vi "process raw data (SubVI).vi"(0 "VISA Refnum in":refnum<visa-resource-name>, 5 "error in (no error)":errorcluster) -> (6 "Raw Data":string, 8 "RSM (Digital)":dbl, 9 "Rain Intensity":dbl(slide) scale=0.0..100.0, 10 "Servo Angle (A)":dbl, 11 "Buzzer Volume (A)":dbl, 12 "Physical Switch State (D)":dbl, 13 "Buzzer Volume":dbl(graph), 14 "VISA Refnum out":refnum<visa-resource-name>, 15 "Servo Angle":dbl(graph), 16 "Rain \nDetected?":bool, 17 "RSM (Analog)":dbl, 18 "Force\nClose?":bool, 19 "error out":errorcluster)   [LabVIEW 2026]
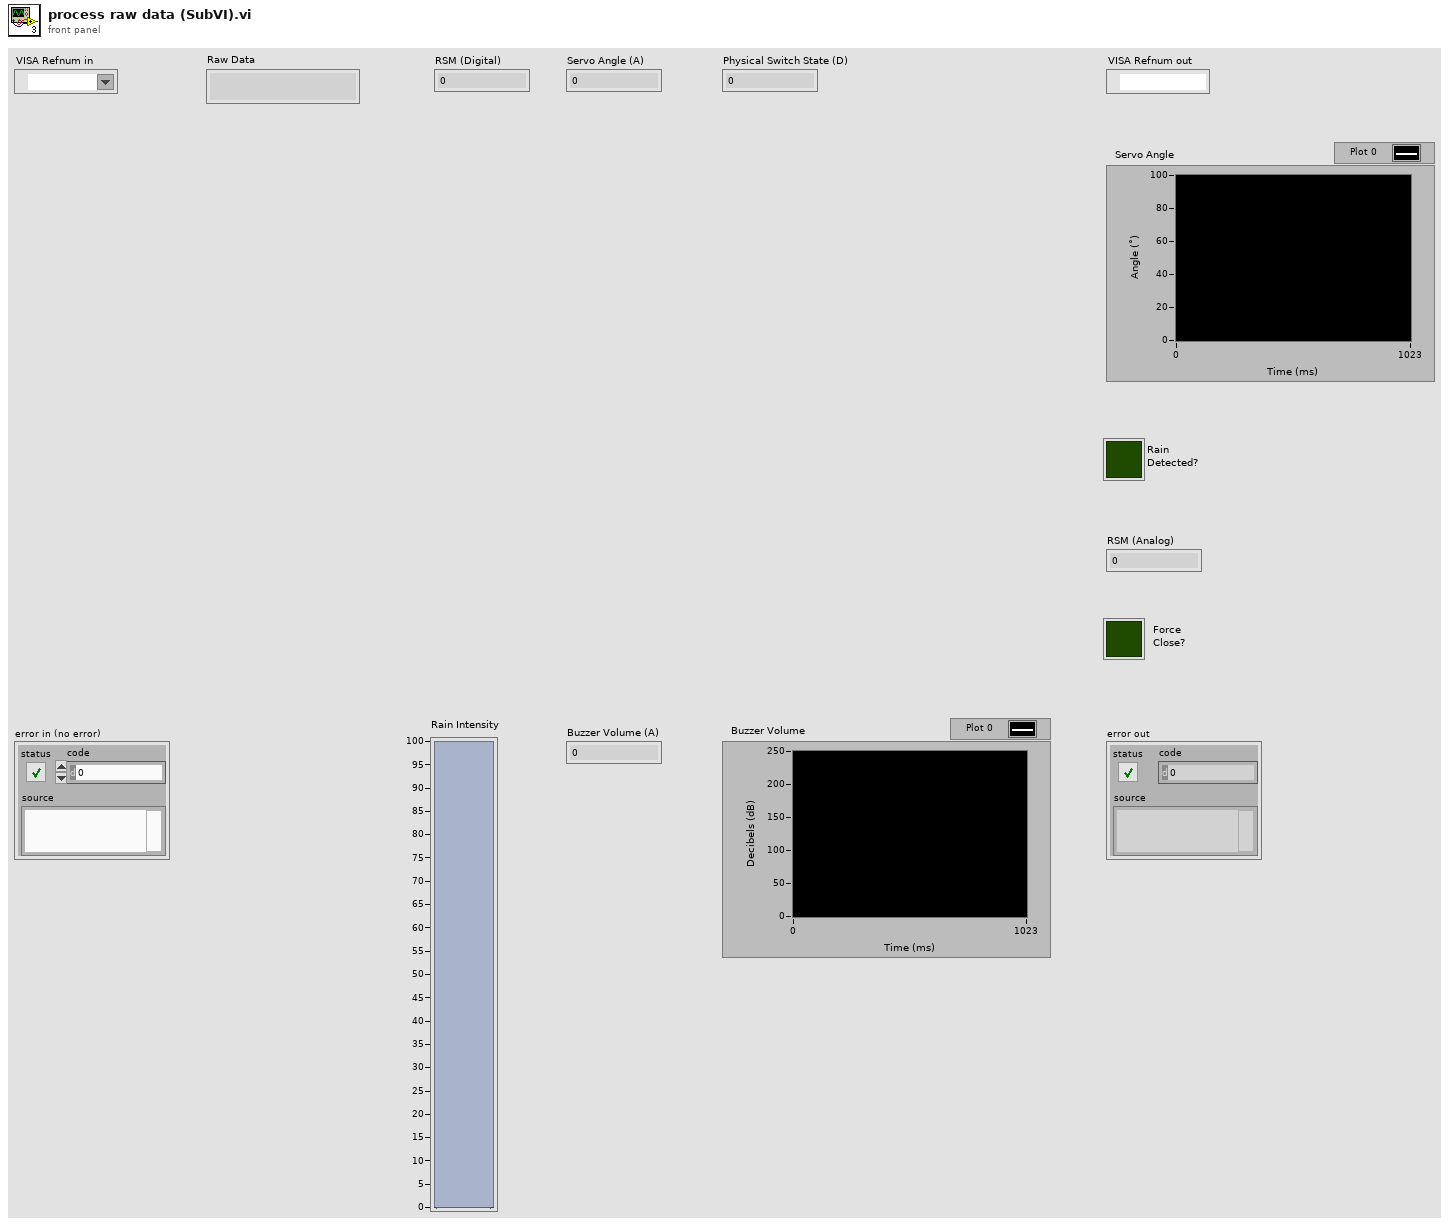
[diagram p1: front panel]
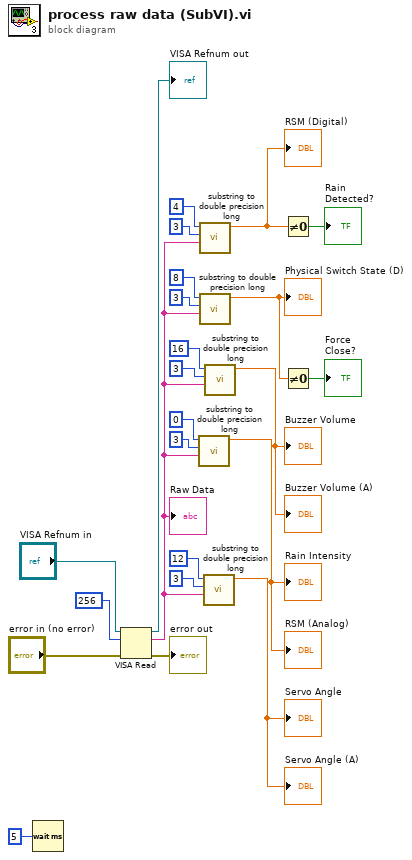
[diagram p0: block diagram]
diagram:
  n1 = Wait (ms)(milliseconds to wait=u32 5) -> ()  [unwired: 1 out]
  n2 = VISA Read(VISA resource name="VISA Refnum in", byte count=u32 256, error in (no error)="error in (no error)") -> (VISA resource name out=→"VISA Refnum out":refnum<visa-resource-name>, read buffer=w16:string, error out=→"error out":errorcluster)  [unwired: 1 out]
  "Raw Data" <- w16
  n3 = call "substring to double precision long.vi"("String Input"=w16, "Length"=3 ("length (rest)"), "Offset"=0 ("offset (0)")) -> ("Numeric"=→"Rain Intensity" →"RSM (Analog)":dbl)  [unwired: 8 in]
  n4 = call "substring to double precision long.vi"("String Input"=w16, "Length"=3 ("length (rest)"), "Offset"=4 ("offset (0)")) -> ("Numeric"=w20:dbl)  [unwired: 8 in]
  "RSM (Digital)" <- w20
  n5 = call "substring to double precision long.vi"("String Input"=w16, "Length"=3 ("length (rest)"), "Offset"=8 ("offset (0)")) -> ("Numeric"=w21:dbl)  [unwired: 8 in]
  "Physical Switch State (D)" <- w21
  n6 = call "substring to double precision long.vi"("String Input"=w16, "Length"=3 ("length (rest)"), "Offset"=12 ("offset (0)")) -> ("Numeric"=→"Servo Angle (A)" →"Servo Angle":dbl)  [unwired: 8 in]
  n7 = call "substring to double precision long.vi"("String Input"=w16, "Length"=3 ("length (rest)"), "Offset"=16 ("offset (0)")) -> ("Numeric"=→"Buzzer Volume (A)" →"Buzzer Volume":dbl)  [unwired: 8 in]
  n8 = Not Equal To 0?(x=w20) -> (x != 0?=→"Rain \nDetected?":bool)
  n9 = Not Equal To 0?(x=w21) -> (x != 0?=→"Force\nClose?":bool)
